vi "Configure MPU.vi"(7 "int on data ready":bool=TRUE, 8 "error in (no error)":errorcluster, 11 "Accelerometer":T1) -> (0 "error out":errorcluster, 3 "Accelerometer out":T1)   [LabVIEW 2013]
doc: "Use this template to build a VI to use as a subVI."
uses:
  AccelerometerSPI.ctl
  <vilib>/ni845x/ni845x.llb/ni845xControl.ctl
  <vilib>/ni845x/ni845x.llb/ni845xSpiConfiguration.ctl
  9250registers.ctl
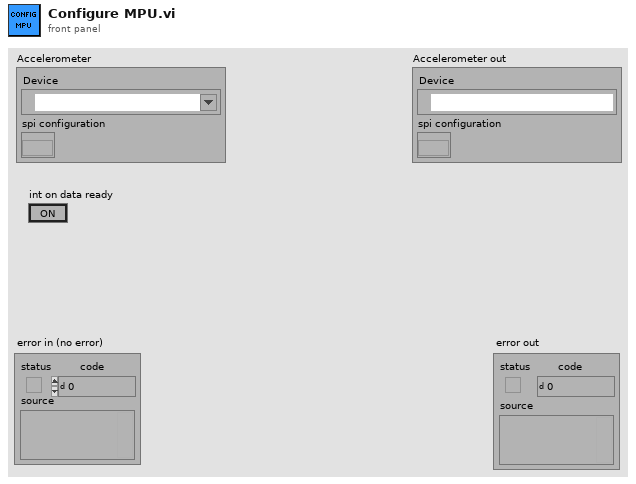
[diagram p1: front panel]
types:
  T1 = typedef "AccelerometerSPI.ctl" = cluster{"Device":T2, "spi configuration":T3}
  T2 = typedef "ni845xControl.ctl" = refnum<k21>
  T3 = typedef "ni845xSpiConfiguration.ctl" = refnum<k20>
  T4 = typedef "9250registers.ctl" = u8
  T5 = cluster{"Device ref out":T2, "spi configuration out":T3}
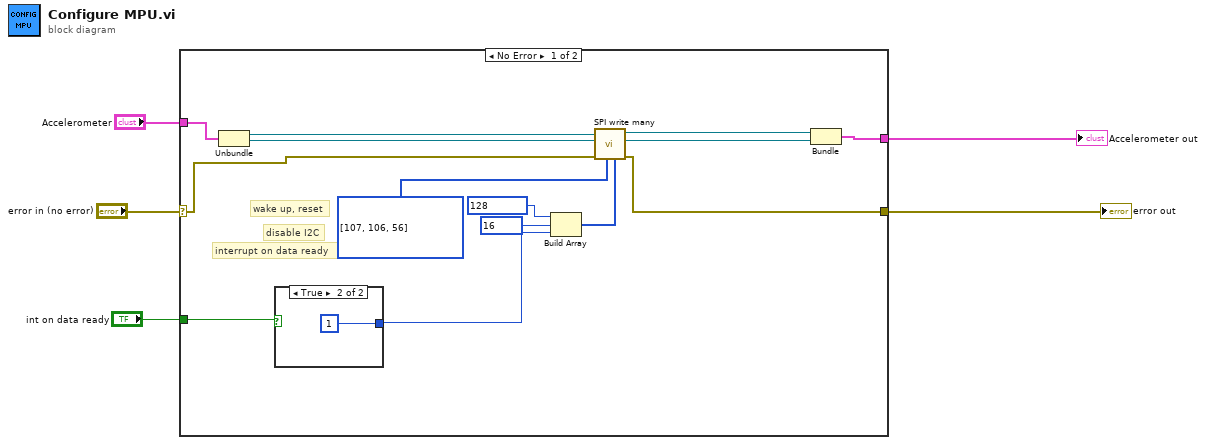
[diagram p0: block diagram]
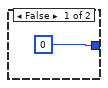
[diagram p2: hidden frame]
diagram:
  n1 = case shown="No Error" "error in (no error)" {
    selector: "error in (no error)" -> [w10 w23]
    tunnel: [w7 w23] -> w4
    tunnel: "Accelerometer" -> [w19 w22]
    tunnel: [w18 w22] -> w2
    tunnel: "int on data ready" -> [w17 _]
    frame No Error {
      w6 = T4[] [107, 106, 56] items=["SELF_TEST_X_GYRO"=0, "SELF_TEST_Y_GYRO"=1, "SELF_TEST_Z_GYRO"=2, "SELF_TEST_X_ACCEL"=13, "SELF_TEST_Y_ACCEL"=14, "SELF_TEST_Z_ACCEL"=15, "XG_OFFSET"=19, "YG_OFFSET"=21, "ZG_OFFSET"=23, "SMPLRT_DIV"=25, "CONFIG"=26, "GYRO_CONFIG"=27, "ACCEL_CONFIG"=28, "ACCEL_CONFIG2"=29, "FIFO_EN"=35, "I2C_MST_CTRL"=36, "I2C_SLV0_ADDR"=37, "I2C_SLV0_REG"=38, "I2C_SLV0_CTRL"=39, "I2C_MST_STATUS"=54, "INT_ENABLE"=56, "INT_STATUS"=58, "ACCEL_XOUT"=59, "ACCEL_YOUT"=61, "ACCEL_ZOUT"=63, "TEMP_OUT"=65, "GYRO_XOUT"=67, "GYRO_YOUT"=69, "GYRO_ZOUT"=71, "EXT_SENS_DATA_00"=73, "I2C_SLV0_D0"=99, "USER_CTRL"=106, "PWR_MGMT_1"=107, "PWR_MGMT_2"=108, "WHO_AM_I"=117, "XA_OFFSET"=119, "YA_OFFSET"=122, "ZA_OFFSET"=125]
      # "disable I2C"
      # "interrupt on data ready"
      # "wake up, reset"
      n2 = Unbundle(w19) -> ("Device"=w12:T2, "spi configuration"=w11:T3)
      n3 = case shown="True" w17 {
        tunnel: [u8 0 u8 1] -> w15
        frame False {
        }
        frame True {
        }
      }
      n4 = Build Array(u8 128, u8 16, w15) -> (w13:u8[])
      n5 = call "SPI write many.vi"("values"=w13, "addresses"=w6, "error in (no error)"=w10, "spi configuration in"=w11, "Device ref in"=w12) -> ("error out"=w7:errorcluster, "spi configuration out"=w8:T3, "Device ref out"=w9:T2)  [unwired: 4 in]
      n6 = Bundle("Device ref out"=w9, "spi configuration out"=w8) -> (w18:T5)  [unwired: 1 in]
    }
    frame Error {
    }
  }
  "error out" <- w4
  "Accelerometer out" <- w2
